vi "4.11.1.vi"() -> ()   [LabVIEW 2018]
panel:
  in  "정지":bool
  in  "a":bool
  out "반복 횟수":i32
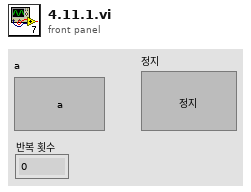
[diagram p1: front panel]
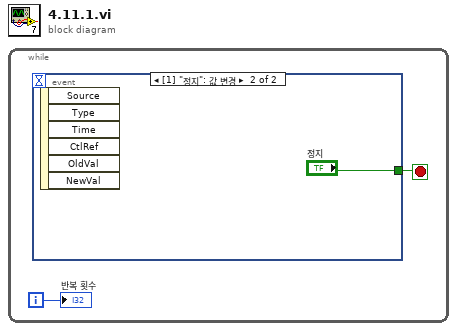
[diagram p0: block diagram]
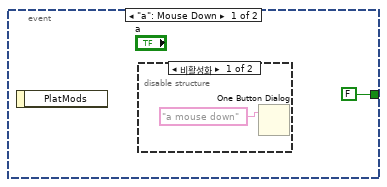
[diagram p2: hidden frame]
diagram:
  n1 = while {
    i -> [w1]
    stop <- w2 stop-if-true
    n2 = event shown="[1] \"정지\": 값 변경" {
      selector: _ -> [_ _]
      dyn-events: _ -> [_ _]
      timeout: _ -> [_ _]
      tunnel: [FALSE ("정지") "정지"] -> w2
      event "a": Mouse Down {
        n3 = event-data() -> ()  [unwired: 1 in, 1 out]
        n4 = disable-structure shown="비활성화" {
          frame Disabled {
            n5 = One Button Dialog(message="a mouse down") -> ()  [unwired: 1 in, 1 out]
          }
          frame Enabled {
          }
        }
      }
      event "정지": Value Change {
        n6 = event-data() -> ()  [unwired: 1 in, 6 out]
      }
    }
    "반복 횟수" <- w1
  }
